vi "gfitsio-open-create-replace-table.vi"(4 "table type (binary)":T1=2 items=["ANY_HDU"=-1, "IMAGE_HDU"=0, "ASCII_TBL"=1, "BINARY_TBL"=2], 5 "prompt (\"Select an HDU\")":string="Select an HDU", 6 "advisory dialog? (display:T)":bool=TRUE, 7 "hdu name (dialog if empty)":string, 8 "error in (no error)":errorcluster, 9 "function (create or replace)":T3(ring)=enum."create or replace", 11 "gfits refnum":T2) -> (0 "error out":errorcluster, 2 "hdu name out":string, 3 "dup gfits refnum":T2)   [LabVIEW 2024, in "gfitsio.lvlib"]
doc: "Opens an existing FITS table HDU, creates a new FITS table HDU, or replaces an existing FITS table HDU, programmatically or interactively using a dialog box. You can optionally specify a dialog prompt."
uses:
  gfitsio.lvlib
  gfitsio-refnum.ctl
  cfitsio-hdutypes.ctl
  gfitsio-error-codes.ctl
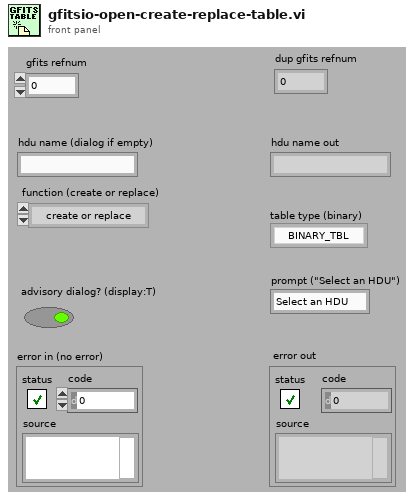
[diagram p1: front panel]
types:
  T1 = typedef "gfitsio.lvlib/cfitsio-hdutypes.ctl" = i32
  T2 = typedef "gfitsio.lvlib/gfitsio-refnum.ctl" = u64
  T3 = enum16{"open", "open or create", "create", "create or replace"}
  T4 = typedef "gfitsio.lvlib/gfitsio-error-codes.ctl" = i32
  T5 = enum16{"Error", "Ok", "Cancel", "Abort", "Retry", "Ignore", "Yes", "No", "Close", "Help", "Disabled"}
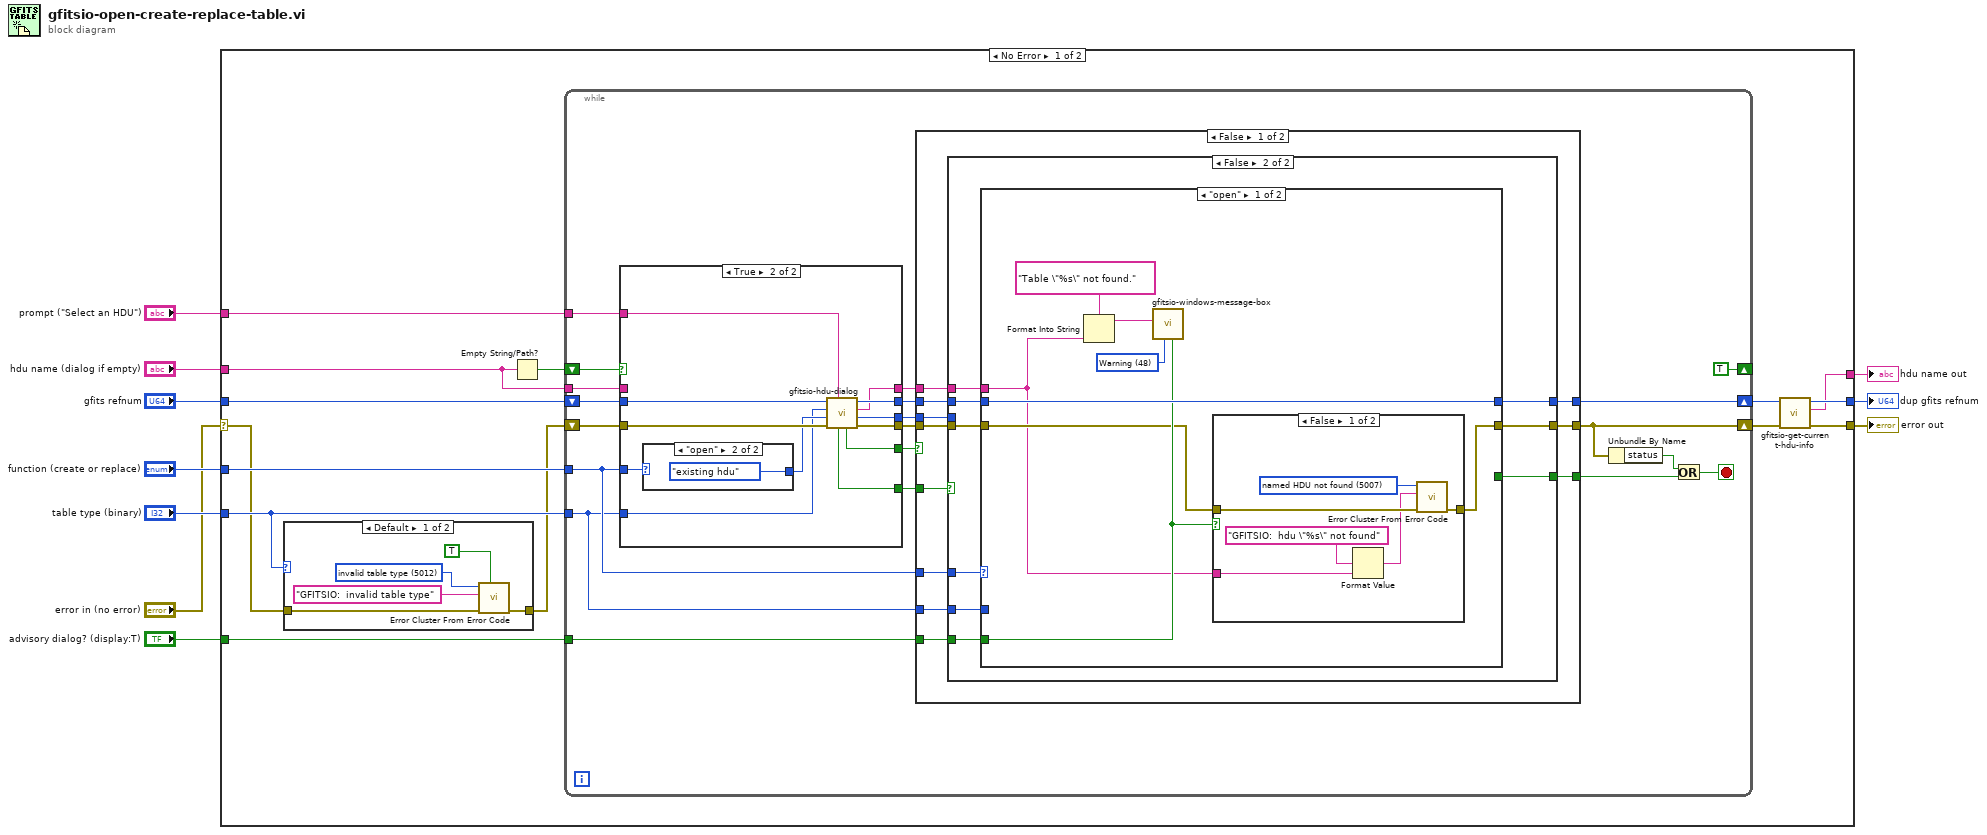
[diagram p0: block diagram]
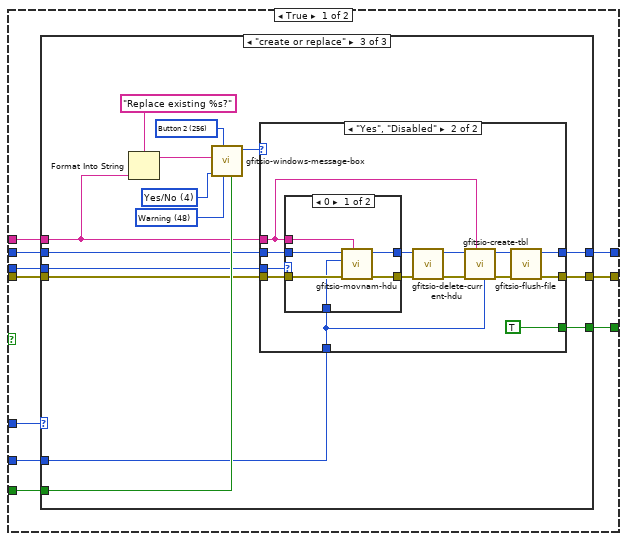
[diagram p3: hidden frame]
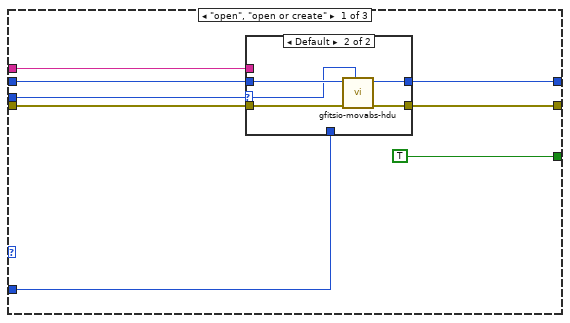
[diagram p4: hidden frame]
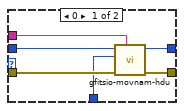
[diagram p5: hidden frame]
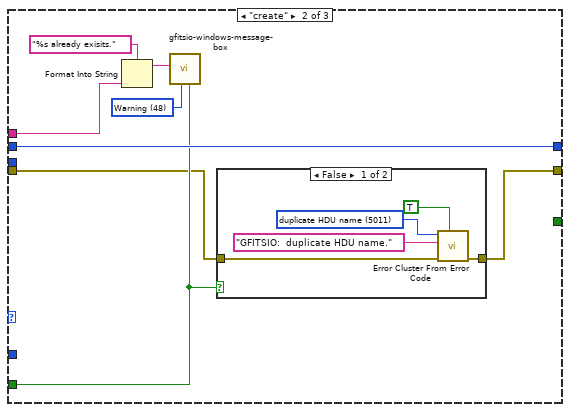
[diagram p6: hidden frame]
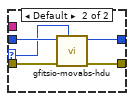
[diagram p9: hidden frame]
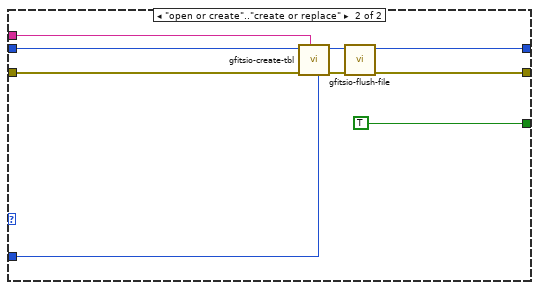
[diagram p11: hidden frame]
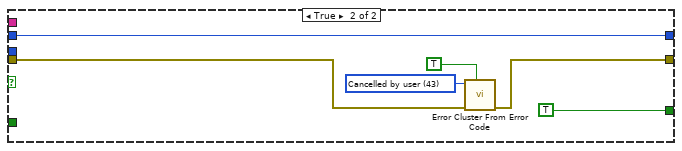
[diagram p12: hidden frame]
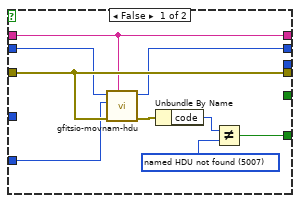
[diagram p13: hidden frame]
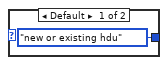
[diagram p14: hidden frame]
diagram:
  n1 = case shown="No Error" "error in (no error)" {
    selector: "error in (no error)" -> [w11 w209]
    tunnel: "advisory dialog? (display:T)" -> [w23 _]
    tunnel: "function (create or replace)" -> [w22 _]
    tunnel: "prompt (\"Select an HDU\")" -> [w21 _]
    tunnel: "hdu name (dialog if empty)" -> [w20 _]
    tunnel: "gfits refnum" -> [w19 w210]
    tunnel: [w16 w209] -> w5
    tunnel: [w15 w210] -> w4
    tunnel: [w14 _] -> w3
    tunnel: "table type (binary)" -> [w13 _]
    frame No Error {
      n2 = case shown="Default" w13 {
        tunnel: w11 -> [w29 w30]
        tunnel: [w28 w30] -> w12
        frame Default {
          w25 = T4 5012 items=["no error"=0, "dimensionality conflict"=5001, "fpixel out of image bounds"=5002, "lpixel out of image bounds"=5003, "increment size larger than image"=5004, "increment must be greater than zero"=5005, "fpixel must specify lower left corner"=5006, "named HDU not found"=5007, "specified row is past the end of the table"=5008, "wrong number of elements for column"=5009, "column is not scalar"=5010, "duplicate HDU name"=5011, "invalid table type"=5012] ("Ring")
          n3 = call <vilib>:"Error Cluster From Error Code.vi"("show call chain? (False)"=TRUE, "error in (no error)"=w29, "error message (\"\")"="GFITSIO:  invalid table type" ("error message (\"\")"), "error code (0)"=w25) -> ("error out"=w28:errorcluster)  [unwired: 5 out]
        }
        frame 1, 2 {
        }
      }
      n4 = Empty String/Path?(string/path=w20) -> (empty?=w24:bool)
      n5 = while {
        tunnel: w13 -> [w33]
        tunnel: w22 -> [w34]
        shift-right: [w43] -> w17
        shift-left: w12 -> [w50]
        shift-right: [w46] -> w18
        shift-left: w19 -> [w49]
        tunnel: w20 -> [w38]
        tunnel: w21 -> [w35]
        tunnel: w23 -> [w32]
        shift-right: [TRUE] -> _
        shift-left: w24 -> [w48]
        stop <- w40 stop-if-true
        n6 = case shown="True" w48 {
          tunnel: [w194 w206] -> w45
          tunnel: [w192 w205] -> w47
          tunnel: w50 -> [w194 w204]
          tunnel: w49 -> [w193 w203]
          tunnel: w33 -> [w188 w195]
          tunnel: w34 -> [_ w202]
          tunnel: [_ w201] -> w44
          tunnel: [w189 w200] -> w39
          tunnel: w38 -> [w187 _]
          tunnel: [w187 w199] -> w37
          tunnel: [_ w198] -> w36
          tunnel: w35 -> [_ w197]
          frame False {
            w186 = T4 5007 items=["no error"=0, "dimensionality conflict"=5001, "fpixel out of image bounds"=5002, "lpixel out of image bounds"=5003, "increment size larger than image"=5004, "increment must be greater than zero"=5005, "fpixel must specify lower left corner"=5006, "named HDU not found"=5007, "specified row is past the end of the table"=5008, "wrong number of elements for column"=5009, "column is not scalar"=5010, "duplicate HDU name"=5011, "invalid table type"=5012] ("Ring")
            n7 = call "gfitsio-movnam-hdu.vi"("extname"=w187, "error in (no error)"=w194, "hdutype (ANY_HDU)"=w188, "gfits refnum"=w193) -> ("error out"=w191:errorcluster, "dup gfits refnum"=w192:T2)  [unwired: 2 in, 4 out]
            n8 = Unbundle By Name(w191) -> ("code"=w190:i32)
            n9 = Not Equal?(x=w190, y=w186) -> (x != y?=w189:bool)
          }
          frame True {
            n10 = case shown="\"open\"" w202 {
              tunnel: [enum32{"existing hdu", "new or existing hdu"}."new or existing hdu" ("select mode (new or existing)") enum32{"existing hdu", "new or existing hdu"}."existing hdu" ("select mode (new or existing)")] -> w196
              frame Default {
              }
              frame "open" {
              }
            }
            n11 = call "gfitsio-hdu-dialog.vi"("prompt (\"Select an HDU\")"=w197, "error in (no error)"=w204, "select mode (new or existing)"=w196, "hdu type (ANY_HDU)"=w195, "gfits refnum"=w203) -> ("error out"=w206:errorcluster, "hdu number (0 if cancelled)"=w198:i32, "hdu name (\"\" if cancelled)"=w199:string, "dup gfits refnum"=w205:T2, "cancelled"=w201:bool, "exists"=w200:bool)  [unwired: 1 out]
          }
        }
        n12 = case shown="False" w44 {
          tunnel: w47 -> [w61 w185]
          tunnel: [w58 w185] -> w46
          tunnel: w45 -> [w60 w181]
          tunnel: [w59 w180] -> w43
          tunnel: [w51 TRUE] -> w41
          tunnel: w39 -> [w57 _]
          tunnel: w37 -> [w54 _]
          tunnel: w36 -> [w53 _]
          tunnel: w34 -> [w56 _]
          tunnel: w33 -> [w55 _]
          tunnel: w32 -> [w52 _]
          frame False {
            n13 = case shown="False" w57 {
              tunnel: w61 -> [w69 w153]
              tunnel: w60 -> [w66 w152]
              tunnel: [w67 w151] -> w59
              tunnel: [w68 w150] -> w58
              tunnel: w56 -> [w71 w155]
              tunnel: w55 -> [w70 w154]
              tunnel: w54 -> [w65 w148]
              tunnel: w53 -> [w64 _]
              tunnel: w52 -> [w63 w149]
              tunnel: [w62 w147] -> w51
              frame True {
                n14 = case shown="\"create or replace\"" w71 {
                  tunnel: w70 -> [w73 _ w105]
                  tunnel: w69 -> [w78 w98 w113]
                  tunnel: [w76 w98 w112] -> w68
                  tunnel: [w77 w91 w110] -> w67
                  tunnel: w66 -> [w79 w92 w111]
                  tunnel: w65 -> [w75 w94 w107]
                  tunnel: w64 -> [w74 _ w106]
                  tunnel: w63 -> [_ w93 w114]
                  tunnel: [TRUE _ w108] -> w62
                  frame "open", "open or create" {
                    n15 = case shown="Default" w74 {
                      selector: w74 -> [_ w86]
                      tunnel: w79 -> [w85 w89]
                      tunnel: w78 -> [w84 w90]
                      tunnel: [w83 w88] -> w77
                      tunnel: [w82 w87] -> w76
                      tunnel: w75 -> [w81 _]
                      tunnel: w73 -> [w80 _]
                      frame 0 {
                        n16 = call "gfitsio-movnam-hdu.vi"("extname"=w81, "error in (no error)"=w85, "hdutype (ANY_HDU)"=w80, "gfits refnum"=w84) -> ("error out"=w83:errorcluster, "dup gfits refnum"=w82:T2)  [unwired: 2 in, 4 out]
                      }
                      frame Default {
                        n17 = call "gfitsio-movabs-hdu.vi"("hdunum"=w86, "error in (no error)"=w89, "gfits refnum"=w90) -> ("error out"=w88:errorcluster, "dup gfits refnum"=w87:T2)  [unwired: 1 in, 6 out]
                      }
                    }
                  }
                  frame "create" {
                    w95 = u32 48 items=["None"=0, "Warning"=48, "Confirmation"=64, "Question"=32, "Error"=16, "User Icon"=128] ("Icon (None)")
                    n18 = Format Into String(format string="%s already exisits.", w94) -> (resulting string=w96:string)  [unwired: 2 in, 1 out]
                    n19 = call "gfitsio-windows-message-box.vi"("enable dialog?"=w93, "Icon (None)"=w95, "Text"=w96) -> ()  [unwired: 4 in, 5 out]
                    n20 = case shown="False" w93 {
                      tunnel: w92 -> [w103 w104]
                      tunnel: [w102 w104] -> w91
                      frame False {
                        w99 = T4 5011 items=["no error"=0, "dimensionality conflict"=5001, "fpixel out of image bounds"=5002, "lpixel out of image bounds"=5003, "increment size larger than image"=5004, "increment must be greater than zero"=5005, "fpixel must specify lower left corner"=5006, "named HDU not found"=5007, "specified row is past the end of the table"=5008, "wrong number of elements for column"=5009, "column is not scalar"=5010, "duplicate HDU name"=5011, "invalid table type"=5012] ("Ring")
                        n21 = call <vilib>:"Error Cluster From Error Code.vi"("show call chain? (False)"=TRUE, "error in (no error)"=w103, "error message (\"\")"="GFITSIO:  duplicate HDU name." ("error message (\"\")"), "error code (0)"=w99) -> ("error out"=w102:errorcluster)  [unwired: 5 out]
                      }
                      frame True {
                      }
                    }
                  }
                  frame "create or replace" {
                    w116 = u32 256 items=["Button 1"=0, "Button 2"=256, "Button 3"=512, "Button 4"=1024] ("Default (Button 1)")
                    w117 = u32 4 items=["Abort/Retry/Ignore"=2, "OK"=0, "OK/Cancel"=1, "Retry/Cancel"=5, "Yes/No"=4, "Yes/No/Cancel"=3] ("Buttons (OK)")
                    w118 = u32 48 items=["None"=0, "Warning"=48, "Confirmation"=64, "Question"=32, "Error"=16, "User Icon"=128] ("Icon (None)")
                    n22 = Format Into String(format string="Replace existing %s?", w107) -> (resulting string=w115:string)  [unwired: 2 in, 1 out]
                    n23 = call "gfitsio-windows-message-box.vi"("enable dialog?"=w114, "Icon (None)"=w118, "Default (Button 1)"=w116, "Buttons (OK)"=w117, "Text"=w115) -> ("Button Selected"=w109:T5)  [unwired: 3 in, 3 out]
                    n24 = case shown="\"Yes\", \"Disabled\"" w109 {
                      tunnel: w113 -> [w121 w134]
                      tunnel: [w121 w124] -> w112
                      tunnel: w111 -> [w120 w133]
                      tunnel: [w120 w123] -> w110
                      tunnel: [_ TRUE] -> w108
                      tunnel: w107 -> [_ w127]
                      tunnel: w106 -> [_ w132]
                      tunnel: w105 -> [_ w122]
                      frame "No", Default {
                      }
                      frame "Yes", "Disabled" {
                        n25 = case shown="0" w132 {
                          selector: w132 -> [_ w142]
                          tunnel: w133 -> [w141 w145]
                          tunnel: w134 -> [w140 w146]
                          tunnel: [w139 w144] -> w131
                          tunnel: [w138 w143] -> w130
                          tunnel: w127 -> [w137 _]
                          tunnel: w122 -> [w136 _]
                          frame 0 {
                            n26 = call "gfitsio-movnam-hdu.vi"("extname"=w137, "error in (no error)"=w141, "hdutype (ANY_HDU)"=w136, "gfits refnum"=w140) -> ("error out"=w139:errorcluster, "dup gfits refnum"=w138:T2)  [unwired: 2 in, 4 out]
                          }
                          frame Default {
                            n27 = call "gfitsio-movabs-hdu.vi"("hdunum"=w142, "error in (no error)"=w145, "gfits refnum"=w146) -> ("error out"=w144:errorcluster, "dup gfits refnum"=w143:T2)  [unwired: 1 in, 6 out]
                          }
                        }
                        n28 = call "gfitsio-delete-current-hdu.vi"("error in (no error)"=w131, "gfits refnum"=w130) -> ("error out"=w128:errorcluster, "dup gfits refnum"=w129:T2)  [unwired: 8 out]
                        n29 = call "gfitsio-create-tbl.vi"("tbltype"=w122, "extname"=w127, "error in (no error)"=w128, "gfits refnum"=w129) -> ("error out"=w126:errorcluster, "dup gfits refnum"=w125:T2)  [unwired: 1 in, 5 out]
                        n30 = call "gfitsio-flush-file.vi"("error in (no error)"=w126, "gfits refnum"=w125) -> ("error out"=w123:errorcluster, "dup gfits refnum"=w124:T2)  [unwired: 8 out]
                      }
                    }
                  }
                }
              }
              frame False {
                n31 = case shown="\"open\"" w155 {
                  tunnel: w154 -> [_ w171]
                  tunnel: w153 -> [w163 w178]
                  tunnel: w152 -> [w158 w179]
                  tunnel: [w157 w173] -> w151
                  tunnel: [w163 w172] -> w150
                  tunnel: w149 -> [w159 _]
                  tunnel: w148 -> [w156 w177]
                  tunnel: [_ TRUE] -> w147
                  frame "open" {
                    w160 = u32 48 items=["None"=0, "Warning"=48, "Confirmation"=64, "Question"=32, "Error"=16, "User Icon"=128] ("Icon (None)")
                    n32 = Format Into String(format string="Table \"%s\" not found.", w156) -> (resulting string=w161:string)  [unwired: 2 in, 1 out]
                    n33 = call "gfitsio-windows-message-box.vi"("enable dialog?"=w159, "Icon (None)"=w160, "Text"=w161) -> ()  [unwired: 4 in, 5 out]
                    n34 = case shown="False" w159 {
                      tunnel: w158 -> [w169 w170]
                      tunnel: [w168 w170] -> w157
                      tunnel: w156 -> [w166 _]
                      frame False {
                        w164 = T4 5007 items=["no error"=0, "dimensionality conflict"=5001, "fpixel out of image bounds"=5002, "lpixel out of image bounds"=5003, "increment size larger than image"=5004, "increment must be greater than zero"=5005, "fpixel must specify lower left corner"=5006, "named HDU not found"=5007, "specified row is past the end of the table"=5008, "wrong number of elements for column"=5009, "column is not scalar"=5010, "duplicate HDU name"=5011, "invalid table type"=5012] ("Ring")
                        n35 = Format Value(format string="GFITSIO:  hdu \"%s\" not found", value (0)=w166) -> (output string=w165:string)  [unwired: 1 out]
                        n36 = call <vilib>:"Error Cluster From Error Code.vi"("error in (no error)"=w169, "error message (\"\")"=w165, "error code (0)"=w164) -> ("error out"=w168:errorcluster)  [unwired: 1 in, 5 out]
                      }
                      frame True {
                      }
                    }
                  }
                  frame "open or create".."create or replace" {
                    n37 = call "gfitsio-create-tbl.vi"("tbltype"=w171, "extname"=w177, "error in (no error)"=w179, "gfits refnum"=w178) -> ("error out"=w175:errorcluster, "dup gfits refnum"=w174:T2)  [unwired: 1 in, 5 out]
                    n38 = call "gfitsio-flush-file.vi"("error in (no error)"=w175, "gfits refnum"=w174) -> ("error out"=w173:errorcluster, "dup gfits refnum"=w172:T2)  [unwired: 8 out]
                  }
                }
              }
            }
          }
          frame True {
            w183 = 43 items=["No error", "Argument error", "Memory is full", "Out of zone", "End of file", "File already open", "Generic file I/O error", "File not found", "File permission error", "Disk is full", "Duplicate path", "Too many files open", "System feature not enabled", "Resource file not found", "Cannot add resource", "Resource not found", "Image not found", "Image memory error", "Pen does not exist", "Config type invalid", "Config token not found", "Config parse error", "Config memory error", "Bad external code format", "Bad external code offset", "External code not present", "Null window", "Destroy window error", "Null menu", "Print aborted", "Bad print record", "Print driver error", "Windows error during printing", "Memory error during printing", "Print dialog error", "Generic print error", "Invalid device refnum", "Device not found", "Device parameter error", "Device unit error", "Cannot open device", "Device call aborted", "Generic error", "Cancelled by user", "Object ID too low", "Object ID too high", "Object not in heap", "Unknown heap", "Unknown object (invalid DefProc)", "Unknown object (DefProc not in table)", "Message out of range", "Invalid (null) method", "Unknown message", "Manager call not supported", "Bad address", "Network operation in progress", "Network operation timed out", "Connection is busy", "Network attribute not supported", "Network error", "Address in use", "System out of memory", "Connection aborted", "Connection refused", "Not connected", "Already connected", "Connection closed", "Initialization error (interapplication manager)", "Bad occurrence", "Wait on unbound occurrence handler", "Occurrence queue overflow", "Datalog type conflict", "Unused", "Unrecognized type (interapplication manager)", "Memory corrupt", "Failed to make temporary DLL", "Old CIN version", "Drag socket not found", "Failed to load drop-object", "Failed to register OLE object", "Failed to release OLE object", "Format specifier type mismatch", "Unknown format specifier", "Too few format specifiers", "Too many format specifiers", "Scan failed", "Newer CIN version", "Error converting to variant", "Runtime menu error", "Password tampered", "Variant attribute not found", "Incompatible variant data type", "Event data is not available", "Event Store is not present", "Occurrence is not found", "Event Queue is not created", "Event info is not available in the type library", "Refnum passed is NULL", "Error retrieving Class GUID", "Error retrieving CoClass GUID", "Error retrieving TypeLib GUID.", "Bad built application magic bytes.", "Specific driver is different from the specific driver associated with the Logical Name.", "There is no session opened to the class driver.", "Max Error", "MAX - Error with config objects", "MAX - Error loading configuration", "MAX - Group not supported", "Singlecast connections can not send to multicast addresses.", "Multicast connections can not send to singlecast addresses.", "Specified IP address not in multicast address range.", "Attempt to write to read-only multicast connection.", "Attempt to read from write-only multicast connection.", "The buffer used to receive a datagram was smaller than the datagram itself"]
            n39 = call <vilib>:"Error Cluster From Error Code.vi"("show call chain? (False)"=TRUE, "error in (no error)"=w181, "error code (0)"=w183) -> ("error out"=w180:errorcluster)  [unwired: 6 out]
          }
        }
        n40 = Unbundle By Name(w43) -> ("status"=w42:bool)
        n41 = Or(x=w42, y=w41) -> (x .or. y?=w40:bool)
      }
      n42 = call "gfitsio-get-current-hdu-info.vi"("error in (no error)"=w17, "gfits refnum"=w18) -> ("error out"=w16:errorcluster, "hdu name"=w14:string, "dup gfits refnum"=w15:T2)  [unwired: 1 in, 6 out]
    }
    frame Error {
    }
  }
  "error out" <- w5
  "dup gfits refnum" <- w4
  "hdu name out" <- w3
